vi "CTR_refDesArray.vi"(0 "DOM document in":refnum<k20>, 5 "StreamCluster":T1={"DAQ_Configs"=[], "CTR_Config"={"CTR refDes"="", "CTR IP Addr"="", "Restart"=FALSE}, "Network_Configs"={"Buffer"=1, "ManagmentRate_Hz"=1000, "StreamRate_Hz"=10, "ConnectionHysterisis"=0, "LoggingRate_Hz"=10}, "ConfigXML_Checksum"=""}, 11 "error in":errorcluster) -> (4 "DOM document out":refnum<k20>, 6 "StreamCluster":T1={"DAQ_Configs"=[], "CTR_Config"={"CTR refDes"="", "CTR IP Addr"="", "Restart"=FALSE}, "Network_Configs"={"Buffer"=1, "ManagmentRate_Hz"=1000, "StreamRate_Hz"=10, "ConnectionHysterisis"=0, "LoggingRate_Hz"=10}, "ConfigXML_Checksum"=""}, 8 "refDesArray":string[](array[string]), 10 "refDes per DAQ":i32[](array[numeric]), 15 "error out":errorcluster={"status"=TRUE, "code"=-2633, "source"="Property Node (arg 1) in NI_XML.lvlib:Get Node Text Content.vi->CTR_ControlNodeConfigs.vi->CTR_ReadXML_Config.vi->CTRnode.vi"})   [LabVIEW 2024]
uses:
  Control/CTR_StreamCluster_TypeDef.ctl
  OneDrive - Embry-Riddle Aeronautical University/Admin/Facilities/TC3/TC3 DAC/Code/RTC_PXIe-Code v1_9_0 CODE/QMH-Architecture/support/Control/streamIO_states.ctl
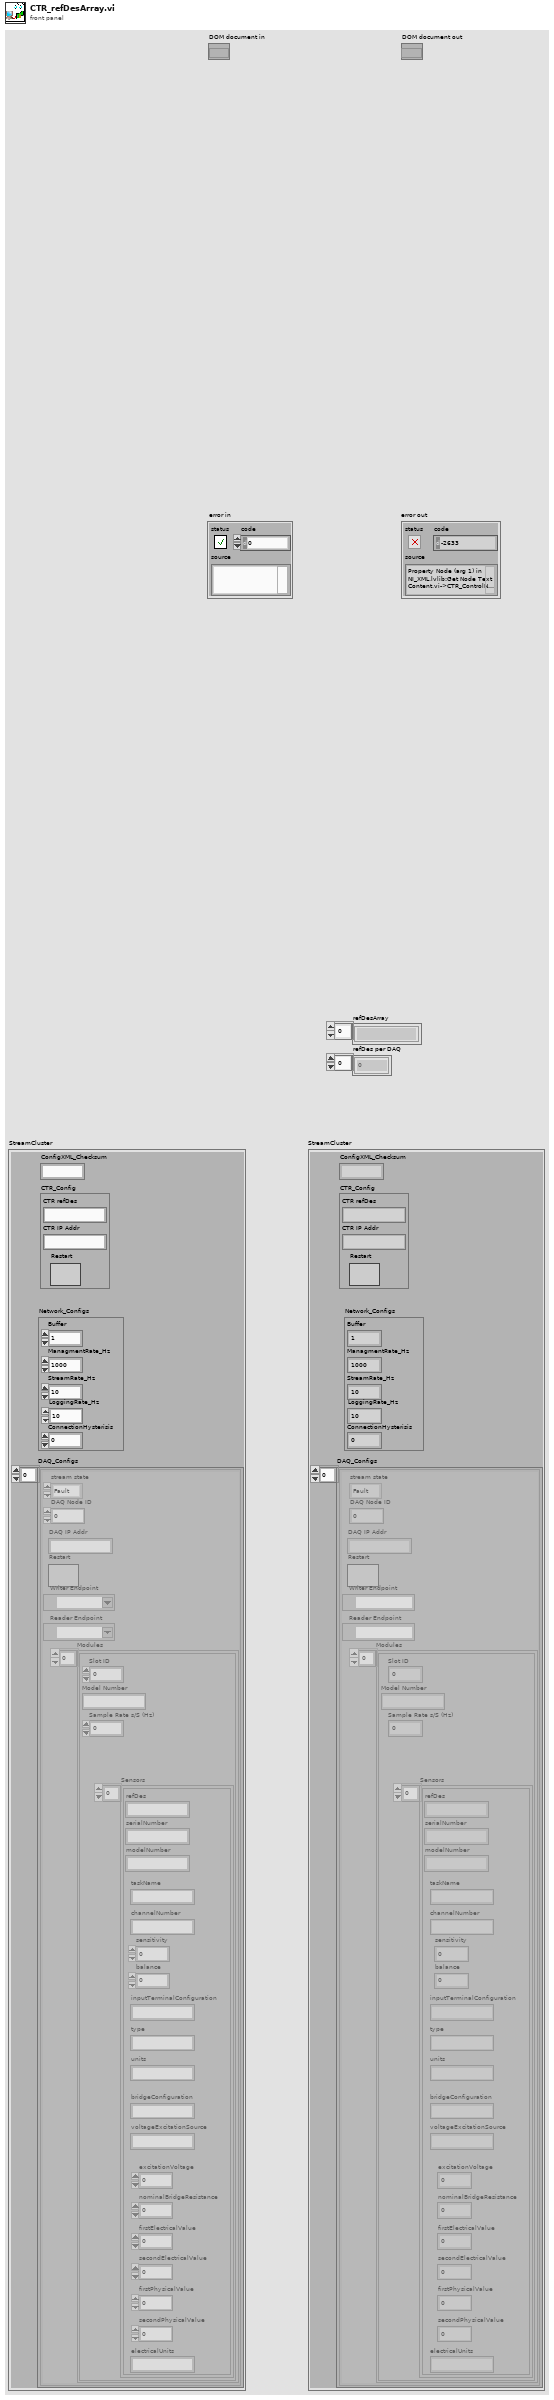
[diagram p1: front panel]
types:
  T1 = typedef "CTR_StreamCluster_TypeDef.ctl" = cluster{"DAQ_Configs":cluster{"stream state":T2, "DAQ Node ID":i32, "Modules":cluster{"Slot ID":i32, "Model Number":string, "Sample Rate s/S (Hz)":dbl, "Sensors":cluster{"refDes":string, "serialNumber":string, "modelNumber":string, "units":string, "balance":dbl, "sensitivity":dbl, "type":string, "inputTerminalConfiguration":string, "channelNumber":string, "taskName":string, "bridgeConfiguration":string, "excitationVoltage":dbl, "voltageExcitationSource":string, "nominalBridgeResistance":dbl, "firstElectricalValue":dbl, "secondElectricalValue":dbl, "firstPhysicalValue":dbl, "secondPhysicalValue":dbl, "electricalUnits":string}[]}[], "DAQ IP Addr":string, "Restart":bool, "Writer Endpoint":refnum<k21>, "Reader Endpoint":refnum<k21>}[], "CTR_Config":cluster{"CTR refDes":string, "CTR IP Addr":string, "Restart":bool}, "Network_Configs":cluster{"Buffer":i32, "ManagmentRate_Hz":i32, "StreamRate_Hz":i32, "ConnectionHysterisis":i32, "LoggingRate_Hz":i32}, "ConfigXML_Checksum":string}
  T2 = typedef "streamIO_states.ctl" = enum16{"Fault", "Initialize", "Stream", "Close"}
  T3 = cluster{"stream state":T2, "DAQ Node ID":i32, "Modules":cluster{"Slot ID":i32, "Model Number":string, "Sample Rate s/S (Hz)":dbl, "Sensors":cluster{"refDes":string, "serialNumber":string, "modelNumber":string, "units":string, "balance":dbl, "sensitivity":dbl, "type":string, "inputTerminalConfiguration":string, "channelNumber":string, "taskName":string, "bridgeConfiguration":string, "excitationVoltage":dbl, "voltageExcitationSource":string, "nominalBridgeResistance":dbl, "firstElectricalValue":dbl, "secondElectricalValue":dbl, "firstPhysicalValue":dbl, "secondPhysicalValue":dbl, "electricalUnits":string}[]}[], "DAQ IP Addr":string, "Restart":bool, "Writer Endpoint":refnum<k21>, "Reader Endpoint":refnum<k21>}[]
  T4 = cluster{"Slot ID":i32, "Model Number":string, "Sample Rate s/S (Hz)":dbl, "Sensors":cluster{"refDes":string, "serialNumber":string, "modelNumber":string, "units":string, "balance":dbl, "sensitivity":dbl, "type":string, "inputTerminalConfiguration":string, "channelNumber":string, "taskName":string, "bridgeConfiguration":string, "excitationVoltage":dbl, "voltageExcitationSource":string, "nominalBridgeResistance":dbl, "firstElectricalValue":dbl, "secondElectricalValue":dbl, "firstPhysicalValue":dbl, "secondPhysicalValue":dbl, "electricalUnits":string}[]}[]
  T5 = cluster{"refDes":string, "serialNumber":string, "modelNumber":string, "units":string, "balance":dbl, "sensitivity":dbl, "type":string, "inputTerminalConfiguration":string, "channelNumber":string, "taskName":string, "bridgeConfiguration":string, "excitationVoltage":dbl, "voltageExcitationSource":string, "nominalBridgeResistance":dbl, "firstElectricalValue":dbl, "secondElectricalValue":dbl, "firstPhysicalValue":dbl, "secondPhysicalValue":dbl, "electricalUnits":string}[]
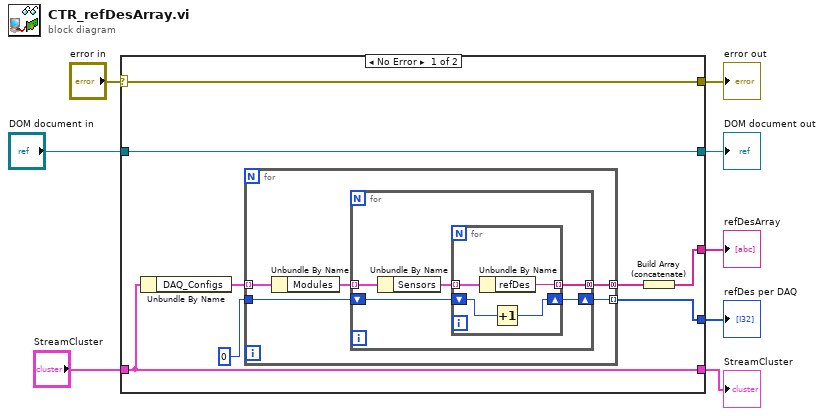
[diagram p0: block diagram]
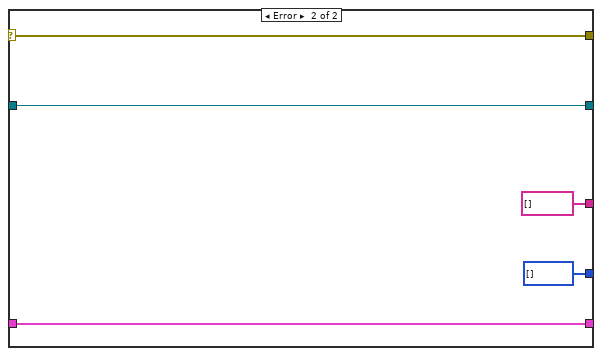
[diagram p2: hidden frame]
diagram:
  n1 = case shown="No Error" "error in" {
    selector: "error in" -> [w15 w35]
    tunnel: [w15 w35] -> w7
    tunnel: "StreamCluster" -> [w16 w34]
    tunnel: [w16 w34] -> w3
    tunnel: "DOM document in" -> [w14 w33]
    tunnel: [w14 w33] -> w5
    tunnel: [w11 string[] []] -> w2
    tunnel: [w9 i32[] []] -> w1
    frame No Error {
      n2 = Unbundle By Name(w16) -> ("DAQ_Configs"=w13:T3)
      n3 = for {
        tunnel: w13 -> [w21] mode=indexing
        tunnel: [w19] -> w12 mode=concatenating
        tunnel: 0 -> [w18]
        tunnel: [w17] -> w9 mode=indexing
        n4 = Unbundle By Name(w21) -> ("Modules"=w20:T4)
        n5 = for {
          tunnel: w20 -> [w26] mode=indexing
          tunnel: [w24] -> w19 mode=concatenating
          shift-right: [w22] -> w17
          shift-left: w18 -> [w23]
          n6 = Unbundle By Name(w26) -> ("Sensors"=w25:T5)
          n7 = for {
            tunnel: w25 -> [w30] mode=indexing
            tunnel: [w29] -> w24 mode=indexing
            shift-right: [w27] -> w22
            shift-left: w23 -> [w28]
            n8 = Unbundle By Name(w30) -> ("refDes"=w29:string)
            n9 = Increment(x=w28) -> (x+1=w27:i32)
          }
        }
      }
      n10 = Build Array (concatenate)(w12) -> (w11:string[])
    }
    frame Error {
    }
  }
  "error out" <- w7
  "DOM document out" <- w5
  "StreamCluster" <- w3
  "refDesArray" <- w2
  "refDes per DAQ" <- w1
